vi "Create.vi"(9 "Alias":string, 10 "Actor":refnum<class "Actor.lvclass">, 11 "Dev Actor in":refnum<class "Dev Actor.lvclass">) -> (3 "Dev Actor out":refnum<class "Dev Actor.lvclass">)   [LabVIEW 2021, in "Dev Actor.lvlib" / "Dev Actor.lvclass"]
uses:
  Dev Actor.lvclass
  <vilib>/jettl/jettl/Actor/Actor/Actor.lvclass
  Dev Actor.lvclass/Dev Actor.ctl
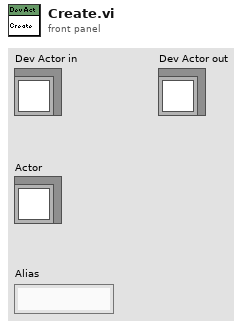
[diagram p1: front panel]
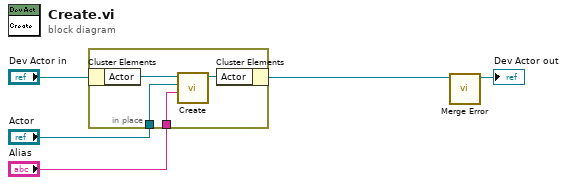
[diagram p0: block diagram]
diagram:
  n1 = in-place {
    in-place-border: "Actor" -> [w6]
    in-place-border: "Alias" -> [w7]
    n2 = in-place-cluster #1("Dev Actor in") -> ("Actor"=w8:refnum<class "Actor.lvclass">)
    n3 = call-dynamic "Create.vi"("Alias"=w7, "Actor"=w6, "Create in"=w8) -> ("Create out"=w9:refnum<class "Actor.lvclass">)  [unwired: 8 in]
    n4 = in-place-cluster #1("Actor"=w9) -> (w2:refnum<class "Dev Actor.lvclass">)
  }
  n5 = call-dynamic "Merge Error.vi"("Dev Actor in"=w2) -> ("Dev Actor out"=→"Dev Actor out":refnum<class "Dev Actor.lvclass">)  [unwired: 10 in]
